vi "test_Add Array Type Cast.vi"(8 "error in (no error)":errorcluster, 11 "TestCase in":refnum<class "Instrument Addon Scripting API Channels Unit Tests.lvclass">) -> (0 "error out":errorcluster, 3 "TestCase out":refnum<class "Instrument Addon Scripting API Channels Unit Tests.lvclass">)   [LabVIEW 2018, in "Instrument Addon Scripting API Channels Unit Tests.lvclass"]
uses:
  Instrument Addon Scripting API Channels Unit Tests.lvclass
  APIs/Scripting API/TypeDefs/Array Type Cast Settings.ctl
  APIs/Scripting API/TypeDefs/Array Element.ctl
  Addon/Addon Shared/Types/Type Cast Type.ctl
  Addon/Addon Shared/Types/Endian.ctl
  Addon/Addon Shared/Types/Protocol Data Type.ctl
  Addon/Addon Shared/Types/Data Channel Type.ctl
  Instrument Addon Scripting API Channels Unit Tests.lvclass/Instrument Addon Scripting API Channels Unit Tests.ctl
  Addon/Addon Shared/SubVIs/Constants.vi
  <vilib>/NI/NI VeriStand Advanced SysDef API/_SubVIs/SysDef.Search.GUID.vi
  <vilib>/NI/NI VeriStand Advanced SysDef API/_SubVIs/SysDef.Search.GUIDs.vi
  APIs/Scripting API/Channels/Create Data Channel - Array - Type Cast.vi
  <vilib>/NI Veristand/Custom Device API/Get Item Property (U16).vi
  <vilib>/NI Veristand/Custom Device API/Get Item Property (String).vi
  <vilib>/addons/_JKI Toolkits/VI Tester/TestCase.llb/TestCase.lvclass
  Instrument Addon Scripting API Test Assets/Instrument Addon Scripting API Test Assets.lvclass
  <vilib>/NI/NI VeriStand Advanced SysDef API/SysDef API/Advanced System Definition.lvlib
  Addon/Addon Shared/Instrument Addon Shared.lvlib
  APIs/Scripting API/Instrument Addon Scripting API.lvlib
  <vilib>/NI Veristand/Custom Device API/Custom Device API.lvlib
  C:/Program Files (x86)/National Instruments/LabVIEW 2018/vi.lib/addons/_JKI Toolkits/VI Tester/TestCase.llb/TestCase.lvclass
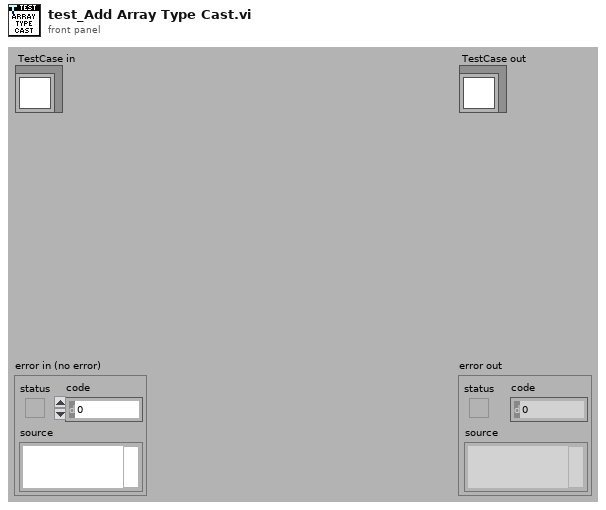
[diagram p1: front panel]
types:
  T1 = typedef "Instrument Addon Scripting API.lvlib/Array Type Cast Settings.ctl" = cluster{"Elements":T2[], "Type":T3, "Endian":T4, "Delimiter":string}
  T2 = typedef "Instrument Addon Scripting API.lvlib/Array Element.ctl" = cluster{"Name":string, "Default Value":dbl, "Units":string}
  T3 = typedef "Instrument Addon Shared.lvlib/Type Cast Type.ctl" = enum16{"DBL", "SGL", "U64", "U32", "U16", "U8", "I64", "I32", "I16", "I8"}
  T4 = typedef "Instrument Addon Shared.lvlib/Endian.ctl" = enum16{"Native", "Little", "Big"}
  T5 = typedef "Instrument Addon Shared.lvlib/Data Channel Type.ctl" = enum16{"Format", "Comparison", "Type Cast", "Enumerated List"}
  T6 = typedef "Instrument Addon Shared.lvlib/Protocol Data Type.ctl" = enum16{"Single Channel", "Array"}
  T7 = typedef "Custom Device API.lvlib/Custom Device Item Ref.ctl" = u64
  T8 = typedef "Advanced System Definition.lvlib/TreeItem.Info.ctl" = cluster{"Name":string, "Description":string, "GUID":string, "Is Channel":bool, "Channel":T9, "Is Waveform":bool, "Waveform":T11}
  T9 = typedef "Custom Device API.lvlib/Custom Device Channel.ctl" = cluster{"Type":T10, "Units":string, "Default Value":dbl, "Faultable":bool, "Scalable":bool}
  T10 = typedef "Custom Device API.lvlib/Custom Device Channel Type.ctl" = enum16{"Input", "Output"}
  T11 = typedef "Custom Device API.lvlib/Custom Device Waveform.ctl" = cluster{"Data Type":T12, "Units":string}
  T12 = typedef "Custom Device API.lvlib/Custom Device Waveform DataType.ctl" = enum16{"Double", "Complex Double"}
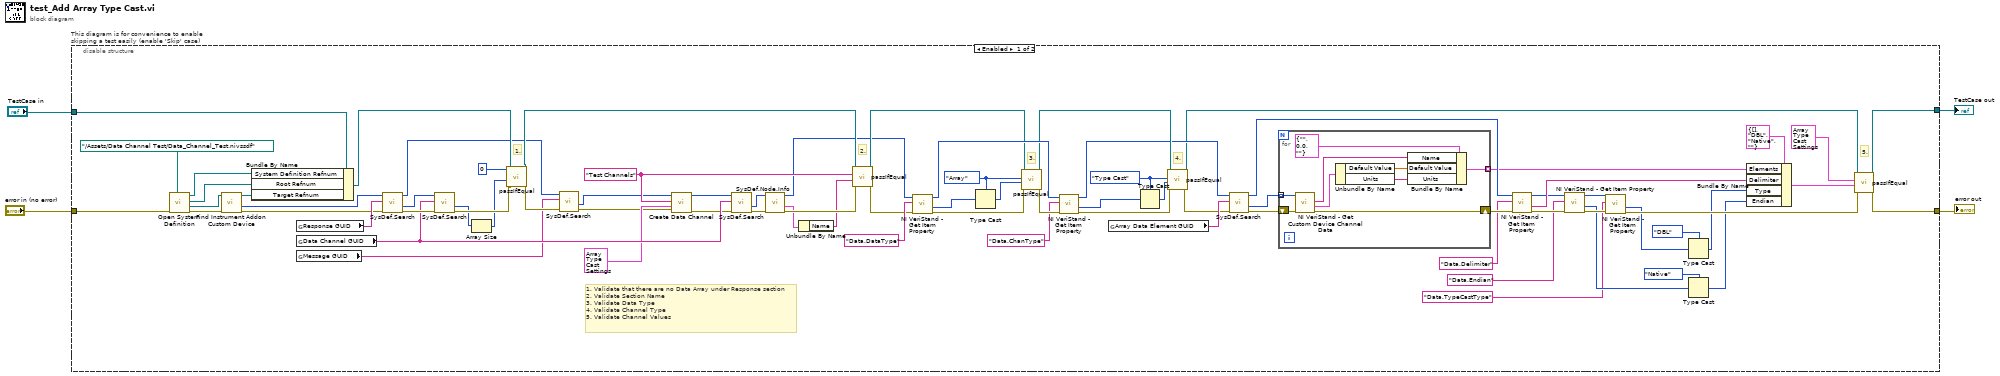
[diagram p0: block diagram]
diagram:
  n1 = disable-structure "This diagram is for convenience to enable skipping a test easily (enable 'Skip' case)" shown="Enabled" {
    disable-tunnel: "TestCase in" -> [w35 w96]
    disable-tunnel: [w57 w94] -> w1
    disable-tunnel: [w58 w95] -> w3
    disable-tunnel: "error in (no error)" -> [w80 w93]
    frame Enabled {
      w14 = Data_Channel_Type."Type Cast" ("Channel Type")
      w19 = Protocol_Data_Type."Array" ("Data Type")
      w69 = "Test Channels" ("Name")
      # "1. Validate that there are no Data Array under Response section\n2. Validate Section Name\n3. Validate Data Type\n4. Validate Channel Type\n5. Validate Channel Values"
      # "4."
      # "3."
      # "5."
      # "2."
      # "1."
      n2 = call "Open System Definition.vi"("error in (no error)"=w80, "System Definition File"=path "../Assets/Data Channel Test/Data_Channel_Test.nivssdf") -> ("error out"=w83:errorcluster, "Target Refnum"=w82:refnum<k24>, "Root Refnum"=w33:refnum<k24>, "System Definition Refnum"=w34:refnum<k24>)  [unwired: 6 in]
      n3 = call "Find Instrument Addon Custom Device.vi"("error in"=w83, "target in"=w82) -> ("error out"=w36:errorcluster, "NodeID"=w79:u64, "target out"=w32:refnum<k24>)  [unwired: 7 in]
      n4 = Bundle By Name(cluster=w35, "System Definition Refnum"=w34, "Root Refnum"=w33, "Target Refnum"=w32) -> (w31:refnum<class "Instrument Addon Scripting API Channels Unit Tests.lvclass">)
      n5 = global read "Constants.vi" "Response GUID"() -> (w78:string)
      n6 = global read "Constants.vi" "Data Channel GUID"() -> (w75:string)
      n7 = global read "Constants.vi" "Message GUID"() -> (w27:string)
      n8 = call-poly <vilib>:"SysDef.Search.vi"("error in (no error)"=w36, "GUID"=w78, "nodeID"=w79) -> ("error out"=w76:errorcluster, "Value out"=w77:u64, "nodeID out"=w26:u64)  [unwired: 5 in, 1 out]
      n9 = call-poly <vilib>:"SysDef.Search.vi"("error in (no error)"=w76, "GUID"=w75, "nodeID"=w77) -> ("error out"=w73:errorcluster, "Values Out"=w72:u64[])  [unwired: 5 in, 2 out]
      n10 = Array Size(array=w72) -> (size(s)=w71:i32)
      n11 = call-dynamic "passIfEqual.vi"("error in (no error)"=w73, "y"=w71, "x"=0 ("size(s)"), "TestCase in"=w31) -> ("error out"=w30:errorcluster, "TestCase out"=w74:refnum<class "Instrument Addon Scripting API Channels Unit Tests.lvclass">)  [unwired: 6 in]
      n12 = call-poly <vilib>:"SysDef.Search.vi"("error in (no error)"=w30, "GUID"=w27, "nodeID"=w26) -> ("error out"=w29:errorcluster, "Value out"=w28:u64)  [unwired: 5 in, 2 out]
      n13 = call-poly "Create Data Channel.vi"("Error In"=w29, "Settings"=T1 {"Elements"=[{"Name"="Wait Time", "Default Value"=2.0, "Units"="ms"}, {"Name"="Rate", "Default Value"=15.0, "Units"="Hz"}], "Type"=enum."I8", "Endian"=enum."Little", "Delimiter"="_"}, "Name"=w69, "Message Refnum In"=w28) -> ("Error Out"=w68:errorcluster, "Message Refnum Out"=w67:T7)  [unwired: 5 in, 1 out]
      n14 = call-poly <vilib>:"SysDef.Search.vi"("error in (no error)"=w68, "GUID"=w75, "nodeID"=w67) -> ("error out"=w66:errorcluster, "Value out"=w65:u64)  [unwired: 5 in, 2 out]
      n15 = call <vilib>:"SysDef.Node.Info.vi"("error in (no error)"=w66, "nodeID"=w65) -> ("error out"=w64:errorcluster, "Item Info"=w63:T8, "nodeID out"=w8:u64)  [unwired: 6 in, 1 out]
      n16 = Unbundle By Name(w63) -> ("Name"=w62:string)
      n17 = call-dynamic "passIfEqual.vi"("error in (no error)"=w64, "y"=w62, "x"=w69, "TestCase in"=w74) -> ("error out"=w9:errorcluster, "TestCase out"=w10:refnum<class "Instrument Addon Scripting API Channels Unit Tests.lvclass">)  [unwired: 6 in]
      n18 = call-poly <vilib>:"NI VeriStand - Get Item Property.vi"("error in (no error)"=w9, "Property Name"="Data.DataType", "Item Ref in"=w8) -> ("error out"=w22:errorcluster, "Value"=w21:u16, "Item Ref out"=w13:T7)  [unwired: 5 in, 1 out]
      n19 = Type Cast(type=w19, x=w21) -> (*(type *) &x=w20:T6)
      n20 = call-dynamic "passIfEqual.vi"("error in (no error)"=w22, "y"=w20, "x"=w19, "TestCase in"=w10) -> ("error out"=w18:errorcluster, "TestCase out"=w7:refnum<class "Instrument Addon Scripting API Channels Unit Tests.lvclass">)  [unwired: 6 in]
      n21 = call-poly <vilib>:"NI VeriStand - Get Item Property.vi"("error in (no error)"=w18, "Property Name"="Data.ChanType", "Item Ref in"=w13) -> ("error out"=w17:errorcluster, "Value"=w16:u16, "Item Ref out"=w6:T7)  [unwired: 5 in, 1 out]
      n22 = global read "Constants.vi" "Array Data Element GUID"() -> (w60:string)
      n23 = Type Cast(type=w14, x=w16) -> (*(type *) &x=w15:T5)
      n24 = call-dynamic "passIfEqual.vi"("error in (no error)"=w17, "y"=w15, "x"=w14, "TestCase in"=w7) -> ("error out"=w11:errorcluster, "TestCase out"=w5:refnum<class "Instrument Addon Scripting API Channels Unit Tests.lvclass">)  [unwired: 6 in]
      n25 = call-poly <vilib>:"SysDef.Search.vi"("error in (no error)"=w11, "GUID"=w60, "nodeID"=w6) -> ("error out"=w61:errorcluster, "Values Out"=w59:u64[], "nodeID out"=w55:u64)  [unwired: 5 in, 1 out]
      n26 = for {
        shift-right: [w84] -> w56
        shift-left: w61 -> [w91]
        tunnel: w59 -> [w92] mode=indexing
        tunnel: [w85] -> w54 mode=indexing
        n27 = call <vilib>:"NI VeriStand - Get Custom Device Channel Data.vi"("error in (no error)"=w91, "Channel Ref in"=w92) -> ("error out"=w84:errorcluster, "Channel"=w88:T9, "Channel Name"=w89:string)  [unwired: 4 in, 3 out]
        n28 = Unbundle By Name(w88) -> ("Default Value"=w86:dbl, "Units"=w87:string)
        n29 = Bundle By Name(cluster=T2 {"Name"="", "Default Value"=0.0, "Units"=""} ("Array Element"), "Name"=w89, "Default Value"=w86, "Units"=w87) -> (w85:T2)
      }
      n30 = call-poly <vilib>:"NI VeriStand - Get Item Property.vi"("error in (no error)"=w56, "Property Name"="Data.Delimiter", "Item Ref in"=w55) -> ("error out"=w47:errorcluster, "Value"=w50:string, "Item Ref out"=w45:T7)  [unwired: 5 in, 1 out]
      n31 = call-poly <vilib>:"NI VeriStand - Get Item Property.vi"("error in (no error)"=w47, "Property Name"="Data.Endian", "Item Ref in"=w45) -> ("error out"=w46:errorcluster, "Value"=w43:u16, "Item Ref out"=w44:T7)  [unwired: 5 in, 1 out]
      n32 = call-poly <vilib>:"NI VeriStand - Get Item Property.vi"("error in (no error)"=w46, "Property Name"="Data.TypeCastType", "Item Ref in"=w44) -> ("error out"=w53:errorcluster, "Value"=w49:u16)  [unwired: 5 in, 2 out]
      n33 = Type Cast(type=Type_Cast_Type."DBL" ("Type"), x=w49) -> (*(type *) &x=w48:T3)
      n34 = Type Cast(type=Endian."Native" ("Endian"), x=w43) -> (*(type *) &x=w42:T4)
      n35 = Bundle By Name(cluster=T1 {"Elements"=[], "Type"=enum."DBL", "Endian"=enum."Native", "Delimiter"=""} ("Settings"), "Elements"=w54, "Delimiter"=w50, "Type"=w48, "Endian"=w42) -> (w25:T1)
      n36 = call-dynamic "passIfEqual.vi"("error in (no error)"=w53, "y"=w25, "x"=T1 {"Elements"=[{"Name"="Wait Time", "Default Value"=2.0, "Units"="ms"}, {"Name"="Rate", "Default Value"=15.0, "Units"="Hz"}], "Type"=enum."I8", "Endian"=enum."Little", "Delimiter"="_"} ("Settings"), "TestCase in"=w5) -> ("error out"=w58:errorcluster, "TestCase out"=w57:refnum<class "Instrument Addon Scripting API Channels Unit Tests.lvclass">)  [unwired: 6 in]
    }
    frame Disabled {
      # "skip test result while test is under development"
      n37 = call <vilib>:"skip.vi"("error in (no error)"=w93, "TestCase in"=w96) -> ("error out"=w95:errorcluster, "TestCase out"=w94:refnum<class "Instrument Addon Scripting API Channels Unit Tests.lvclass">)  [unwired: 8 in]
    }
  }
  "error out" <- w3
  "TestCase out" <- w1
